vi "TSM SSC Digital Get Site Pass Fail.vi"(0 "Digital TSM In":T1, 11 "error in":errorcluster) -> (4 "Digital TSM Out":T1, 6 "Per-Site Pass":bool[](array[boolean]), 15 "error out":errorcluster)   [LabVIEW 2019]
doc: "Returns per-site pass/fail results for sites connected to the specified pin(s) and pin group(s)."
uses:
  TSM/TSM SSC Digital.ctl
  <vilib>/NI_TestStand_SemiconductorModule/NI_TestStand_Semiconductor_Module.lvlibp/PinMap/Digital Pattern/PinQueryContext/DigitalPatternPinQueryContext.lvclass
  SSC Digital/SSC Digital.ctl
  ce1d78c3-842d-4f0e-ad5f-1c357daba0dc.vi
  Shared SubVIs/Site List to Site Numbers.vi
  Shared SubVIs/Trim Whitespace [Inlined].vi
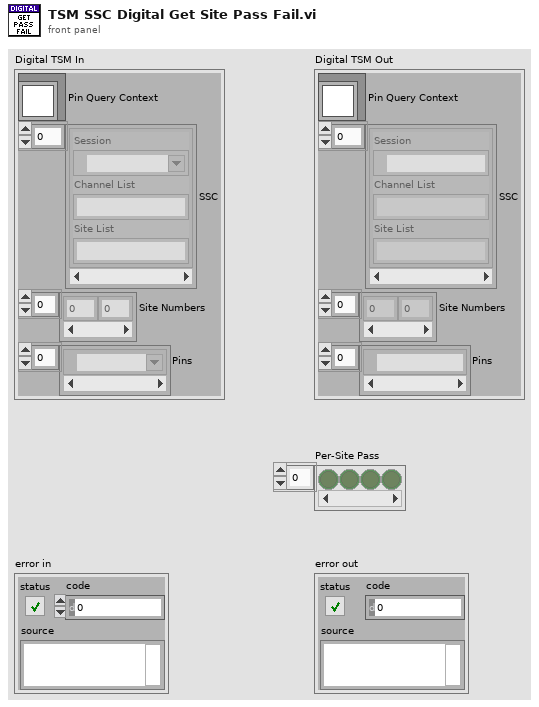
[diagram p1: front panel]
types:
  T1 = typedef "TSM SSC Digital.ctl" = cluster{"Pin Query Context":refnum<class "DigitalPatternPinQueryContext.lvclass">, "SSC":T2[], "Site Numbers":i32[], "Pins":tag[]}
  T2 = typedef "SSC Digital.ctl" = cluster{"Session":refnum<k15>, "Channel List":string, "Site List":string}
  T3 = typedef "Digital 1D Location Array in a Cluster.ctl" = cluster{"Digital 1D Location Array":i32[]}
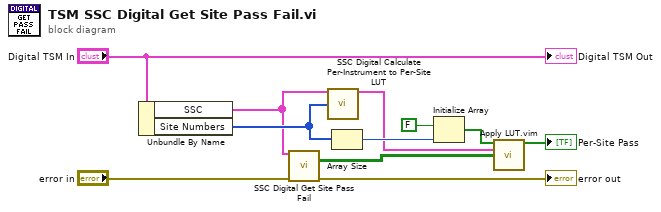
[diagram p0: block diagram]
diagram:
  n1 = Unbundle By Name("Digital TSM In") -> ("SSC"=w1:T2[], "Site Numbers"=w10:i32[])
  n2 = call "SSC Digital Get Site Pass Fail.vi"("Digital SSC in"=w1, "error in"="error in") -> ("Per-Instrument Pass"=w11:bool[][], "error out"=→"error out":errorcluster)  [unwired: 11 in, 1 out]
  n3 = call "SSC Digital Calculate Per-Instrument to Per-Site LUT.vi"("Digital SSC In"=w1, "Sites"=w10) -> ("Per-Instrument to Per-Site LUT"=w3:T3[])  [unwired: 13 in]
  n4 = Array Size(array=w10) -> (size(s)=w9:i32)
  n5 = Initialize Array(FALSE, w9) -> (w7:bool[])
  n6 = call "Apply LUT.vim"("Initialized Array"=w7, "LUT"=w3, "Results to Apply LUT to"=w11) -> ("Array Out"=→"Per-Site Pass":bool[])  [unwired: 12 in]
  "Digital TSM Out" <- "Digital TSM In"
